vi "ClusterToColor.vi"(8 "error in (no error)":errorcluster, 11 "cluster elements info":variant[](array[variant])) -> (0 "error out":errorcluster, 1 "Type":string, 2 "ItemSyms":i32, 3 "Color":u32(colorbox))   [LabVIEW 2020, in "BlueVariantView.lvlib"]
uses:
  BlueVariantView.lvlib
  <vilib>/Utility/Data Type/NI_Data Type.lvlib
  Symbol.ctl
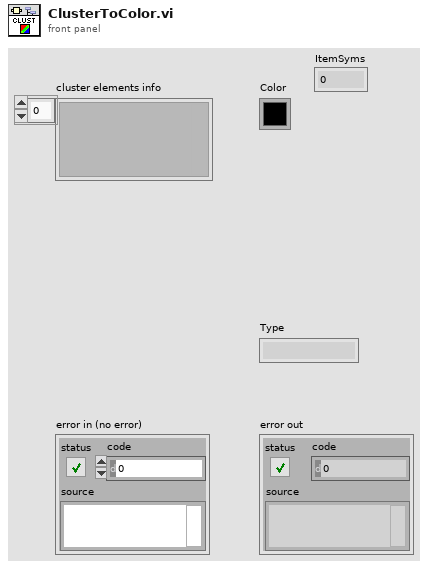
[diagram p1: front panel]
types:
  T1 = typedef "BlueVariantView.lvlib/Symbol.ctl" = enum16{"None", "Cluster-brown", "Cluster-yellow", "Cluster-black", "Cluster-pink", "Array", "Float", "Int", "Bool", "String", "Enum", "Object", "Map", "Set", "Refnum", "Variant", "Path", "Picture", "Waveform", "Timestamp", "Digital Waveform", "Fixed Point"}
  T2 = typedef "NI_Data Type.lvlib/Data Type.ctl" = enum8{"Invalid Type", "Void", "I8", "I16", "I32", "I64", "U8", "U16", "U32", "U64", "Single Float", "Double Float", "Extended Float", "Single Complex", "Double Complex", "Extended Complex", "Enum U8", "Enum U16", "Enum U32", "Enum U64", "Single Float With Unit", "Double Float With Unit", "Extended Float With Unit", "Single Complex with Unit", "Double Complex with Unit", "Extended Complex with Unit", "Boolean", "String", "Path", "Picture", "Tag", "Array", "Cluster", "Variant", "LV Variant", "Waveform", "Timestamp", "Digital Waveform", "Digital Data", "ExpressData", "Refnum", "External Data", "VI", "Poly VI", "LabVIEW Class Instance", "Fixed Point", "Set Collection", "Map Collection"}
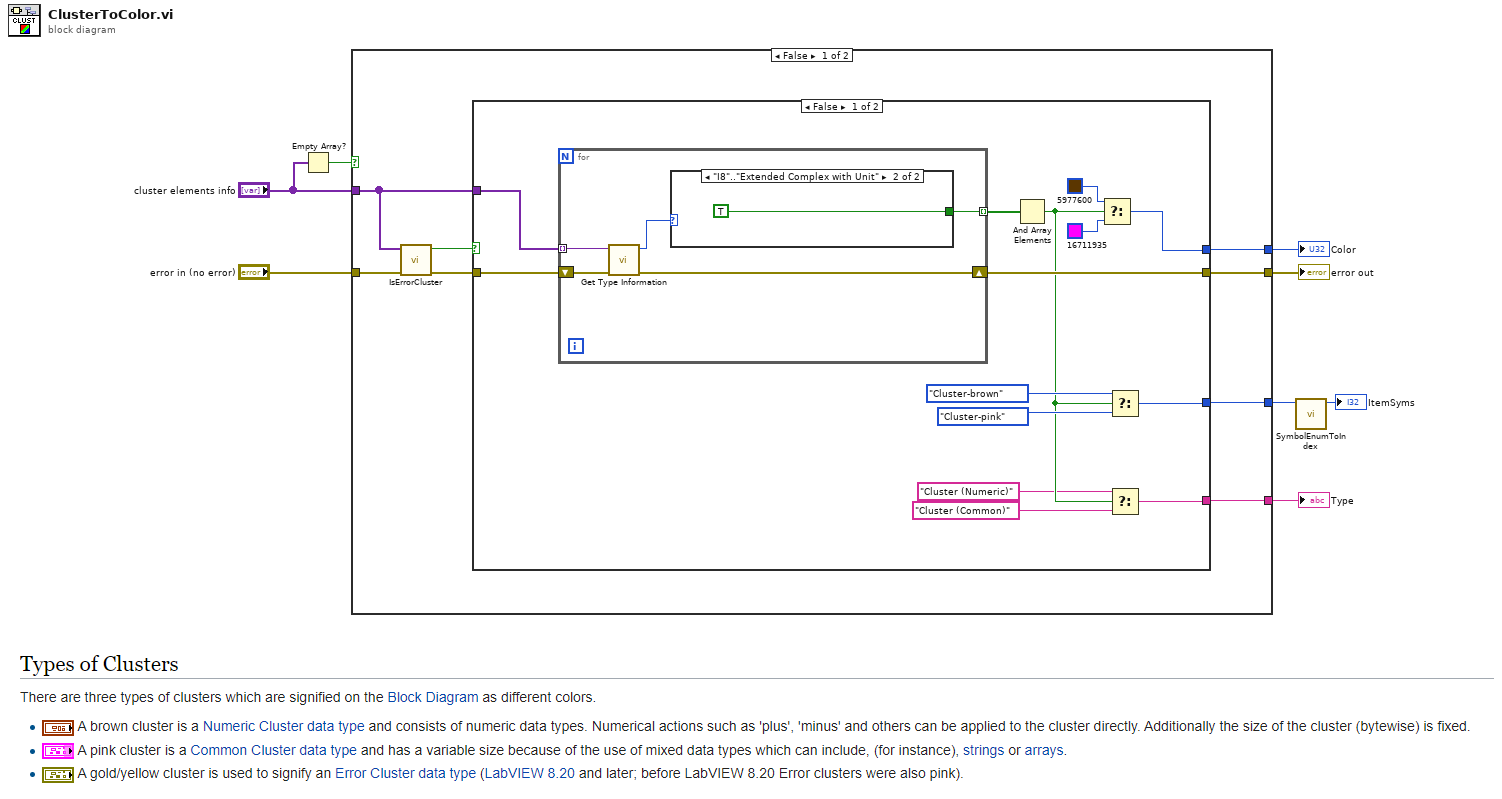
[diagram p0: block diagram]
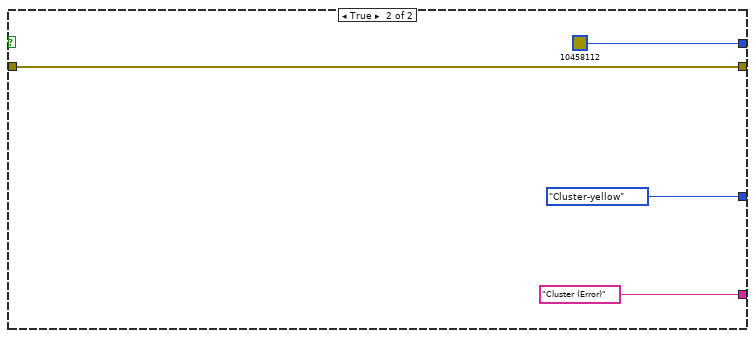
[diagram p3: hidden frame]
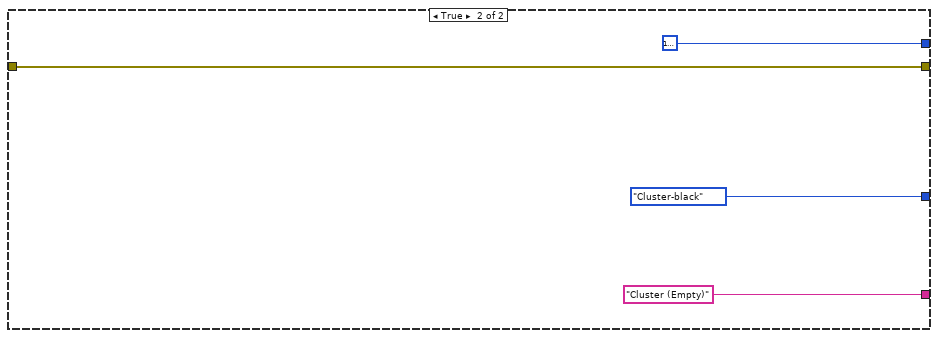
[diagram p4: hidden frame]
diagram:
  n1 = Empty Array?(array="cluster elements info") -> (empty?=w4:bool)
  n2 = case shown="False" w4 {
    tunnel: "error in (no error)" -> [w12 w43]
    tunnel: [w16 w43] -> w7
    tunnel: [w15 u32 16777222] -> w8
    tunnel: [w14 Symbol."Cluster-black" ("Symbol")] -> w2
    tunnel: [w13 "Cluster (Empty)" ("Type")] -> w6
    tunnel: "cluster elements info" -> [w11 _]
    frame False {
      n3 = call "IsErrorCluster.vi"("error in (no error)"=w12, "cluster elements info"=w11) -> ("error out"=w10:errorcluster, "IsErrClust?"=w9:bool)  [unwired: 8 in]
      n4 = case shown="False" w9 {
        tunnel: [w30 w39] -> w16
        tunnel: [w26 u32 10458112] -> w15
        tunnel: [w23 Symbol."Cluster-yellow" ("Symbol")] -> w14
        tunnel: [w20 "Cluster (Error)" ("Type")] -> w13
        tunnel: w11 -> [w18 _]
        tunnel: w10 -> [w17 w39]
        frame False {
          n5 = for {
            tunnel: w18 -> [w35] mode=indexing
            shift-right: [w33] -> w30
            shift-left: w17 -> [w34]
            tunnel: [w31] -> w29 mode=indexing
            n6 = call <vilib>:"Get Type Information.vi"("error in (no error)"=w34, "variant"=w35) -> ("error out"=w33:errorcluster, "type"=w32:T2)  [unwired: 5 in, 3 out]
            n7 = case shown="\"I8\"..\"Extended Complex with Unit\"" w32 {
              tunnel: [_ TRUE] -> w31
              frame Default {
              }
              frame "I8".."Extended Complex with Unit" {
              }
            }
          }
          n8 = And Array Elements(Boolean array=w29) -> (logical AND=w22:bool)
          n9 = Select(t=u32 5977600, s=w22, f=u32 16711935) -> (s? t:f=w26:u32)
          n10 = Select(t=Symbol."Cluster-brown" ("Symbol"), s=w22, f=Symbol."Cluster-pink" ("Symbol")) -> (s? t:f=w23:T1)
          n11 = Select(t="Cluster (Numeric)" ("Type"), s=w22, f="Cluster (Common)" ("Type")) -> (s? t:f=w20:string)
        }
        frame True {
        }
      }
    }
    frame True {
    }
  }
  "error out" <- w7
  "Color" <- w8
  "Type" <- w6
  n12 = call "SymbolEnumToIndex.vi"("symbol enum"=w2) -> ("ItemSyms"=→"ItemSyms":i32)  [unwired: 10 in]
